vi "Remove Invalid Scalars.vi"(8 "error in (no error)":errorcluster, 11 "invalid scalar data channels":T1[](array[typedef]) {"Item Ref" format="%.0x"}) -> (0 "error out":errorcluster)   [LabVIEW 2018, in "FPGA Addon System Explorer.lvlib"]
uses:
  FPGA Addon System Explorer.lvlib
  Types/Output Scalar.ctl
  Addon Shared/Types/Data Type.ctl
  <vilib>/NI Veristand/Custom Device API/Custom Device Item Ref.ctl
  <vilib>/NI Veristand/Custom Device API/Custom Device API.lvlib
  Addon Shared/FPGA Addon Shared.lvlib
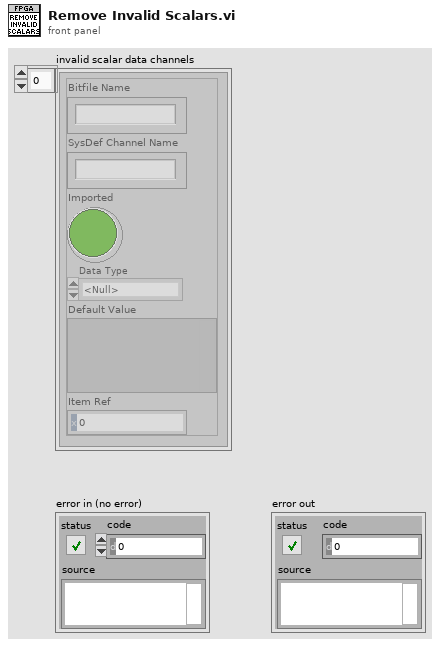
[diagram p1: front panel]
types:
  T1 = typedef "FPGA Addon System Explorer.lvlib/Output Scalar.ctl" = cluster{"Bitfile Name":string, "SysDef Channel Name":string, "Imported":bool, "Data Type":T2, "Default Value":variant, "Item Ref":T3}
  T2 = typedef "FPGA Addon Shared.lvlib/Data Type.ctl" = enum8{"<Null>", "I8", "I16", "I32", "I64", "U8", "U16", "U32", "U64", "SGL", "Boolean", "Analog PWM In Settings", "Analog PWM In", "Digital PWM In Settings", "Digital PWM In", "Digital PWM Out", "Sine Out", "FXP+/-24.5", "FXP+/-16.5", "FXP+/-32.8", "FXP+/-64.32", "FXP+/-16.7", "FXP+/-20.5", "FXP+/-27.5", "FXP+/-32.16", "FXP+16.3", "FXP+18.3", "Digital Static In", "Digital Static Out", "Digital Static In Settings", "Digital WSS Out", "Quad Encoder Settings", "Quad Encoder In", "Group"}
  T3 = typedef "Custom Device API.lvlib/Custom Device Item Ref.ctl" = u64
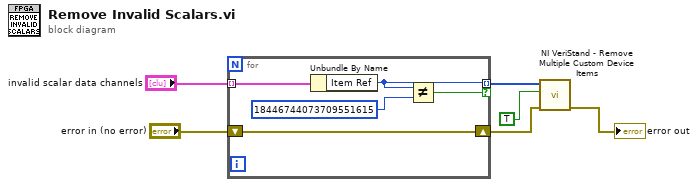
[diagram p0: block diagram]
diagram:
  n1 = for {
    tunnel: "invalid scalar data channels" -> [w11] mode=indexing
    shift-right: [w10] -> w3
    shift-left: "error in (no error)" -> [w10]
    tunnel: [w8] -> w1 mode=indexing if=w7
    n2 = Unbundle By Name(w11) -> ("Item Ref"=w8:T3)
    n3 = Not Equal?(x=w8, y=T3 18446744073709551615) -> (x != y?=w7:bool)
  }
  n4 = call <vilib>:"NI VeriStand - Remove Multiple Custom Device Items.vi"("error in (no error)"=w3, "Force Delete (F)"=TRUE, "Item Refs in"=w1) -> ("error out"=→"error out":errorcluster)  [unwired: 7 in, 1 out]
